vi "NC file to string array.vi"(11 "Path":path=path "C:/Users/Public/Documents/National Instruments/CNC/G-code interperter/G-code.txt") -> (1 "Has Code?":bool, 3 "Code":string[][](array[string]))   [LabVIEW 2011]
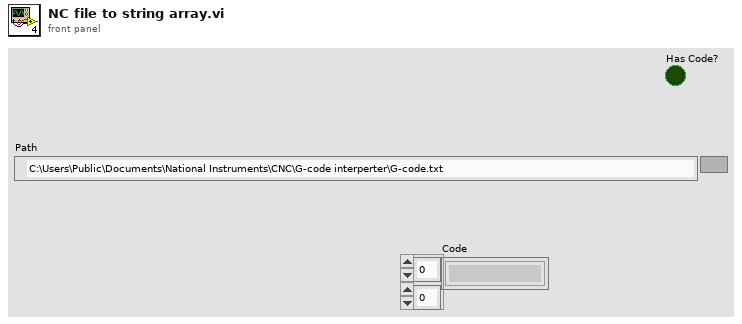
[diagram p1: front panel]
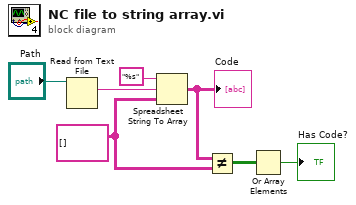
[diagram p0: block diagram]
diagram:
  w3 = string[][] []
  n1 = Read from Text File(file (use dialog)="Path") -> (text=w6:string)  [unwired: 3 in, 3 out]
  n2 = Spreadsheet String To Array(format string="%s", spreadsheet string=w6, array type (2D Dbl)=w3) -> (array=w4:string[][])  [unwired: 1 in]
  "Code" <- w4
  n3 = Not Equal?(x=w4, y=w3) -> (x != y?=w2:bool[][])
  n4 = Or Array Elements(Boolean array=w2) -> (logical OR=→"Has Code?":bool)
